vi "aal_moving average with decimation by order (complex input) (No State).vi"(6 "Reset":bool, 7 "aal_moving average with decimation by order (complex input) state in":T1, 10 "N":i32=1, 11 "x":cdb[](array[numeric]) format="%_6g") -> (3 "y":cdb[](array[numeric]) format="%_6g", 5 "aal_moving average with decimation by order (complex input) state out":T1)   [LabVIEW 2024, in "NI_AALPro.lvlib"]
uses:
  NI_AALPro.lvlib
  <resource>/lvanlys.dll
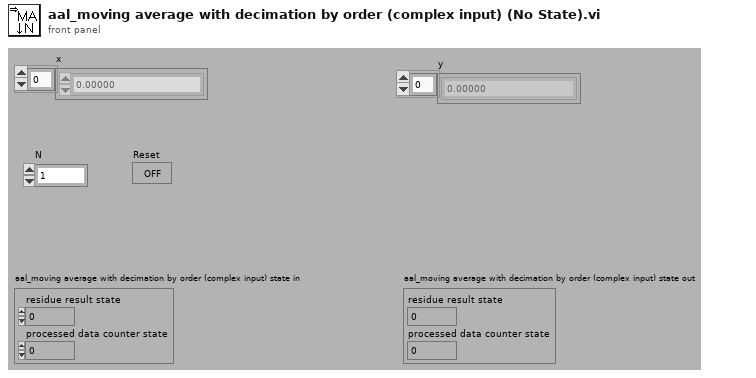
[diagram p1: front panel]
types:
  T1 = cluster{"residue result state":cdb, "processed data counter state":i32}
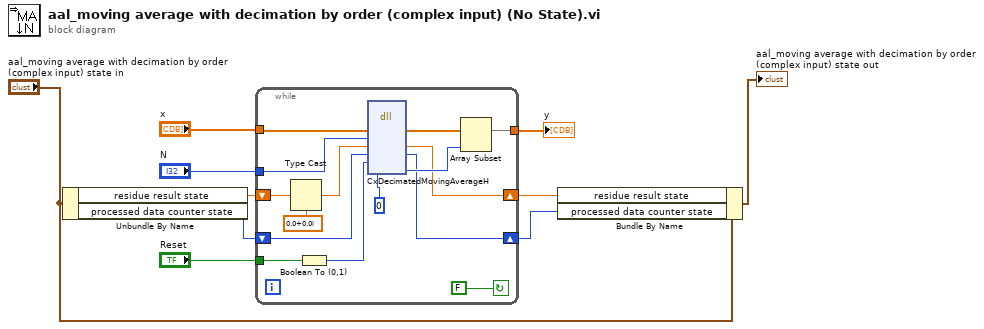
[diagram p0: block diagram]
diagram:
  n1 = Unbundle By Name("aal_moving average with decimation by order (complex input) state in") -> ("residue result state"=w3:cdb, "processed data counter state"=w2:i32)
  n2 = while {
    tunnel: [w22] -> w8
    tunnel: "N" -> [w20]
    tunnel: "Reset" -> [w25]
    tunnel: "x" -> [w24]
    shift-left: w2 -> [w15]
    shift-right: [w13] -> w4
    shift-left: w3 -> [w19]
    shift-right: [w14] -> w5
    stop <- FALSE continue-if-true
    n3 = Type Cast(type=cdb 0.0+0.0i, x=w19) -> (*(type *) &x=w12:cdb)
    n4 = Boolean To (0,1)(Boolean=w25) -> (0, 1=w18:i16)
    n5 = dll-call lib="C:/Program Files (x86)/National Instruments/LabVIEW 2024/resource/lvanlys.*" fn="CxDecimatedMovingAverageH"("xH"=w24, "N"=w20, "stateH"=w12, "cnt"=w15, "reset"=w18, "out_len"=0 ("yH")) -> ("xH"=w23:cdb[], "stateH"=w14:cdb, "cnt"=w13:i32, "out_len"=w16:i32)  [unwired: 6 in, 2 out]
    n6 = Array Subset(array=w23, length=w16) -> (w22:cdb[])  [unwired: 1 in]
  }
  "y" <- w8
  n7 = Bundle By Name(cluster="aal_moving average with decimation by order (complex input) state in", "residue result state"=w5, "processed data counter state"=w4) -> (→"aal_moving average with decimation by order (complex input) state out":T1)
